vi "ReadDiagram.vi"(1 "reference":refnum<vi>) -> (0 "Diagram":T5)   [LabVIEW 2013]
uses:
  <vilib>/Utility/miscctls.llb/LVBoundsTypeDef.ctl
  <vilib>/Utility/miscctls.llb/LVPositionTypeDef.ctl
  <vilib>/Utility/miscctls.llb/LVRectTypeDef.ctl
  <vilib>/Utility/miscctls.llb/LVBreakpointStatusEnum.ctl
panel:
  out "error out 24":errorcluster
  out "error out 23":errorcluster
  out "error out 22":errorcluster
  out "error out 21":errorcluster
  out "error out 20":errorcluster
  out "error out 19":errorcluster
  out "error out 18":errorcluster
  out "error out 17":errorcluster
  out "error out 16":errorcluster
  out "error out 15":errorcluster
  out "error out 14":errorcluster
  out "error out 13":errorcluster
  out "error out 12":errorcluster
  out "error out 11":errorcluster
  out "error out 10":errorcluster
  out "error out 9":errorcluster
  out "error out 8":errorcluster
  out "error out 7":errorcluster
  out "error out 6":errorcluster
  out "error out 5":errorcluster
  out "error out 4":errorcluster
  out "error out 3":errorcluster
  out "error out 2":errorcluster
  out "error out":errorcluster
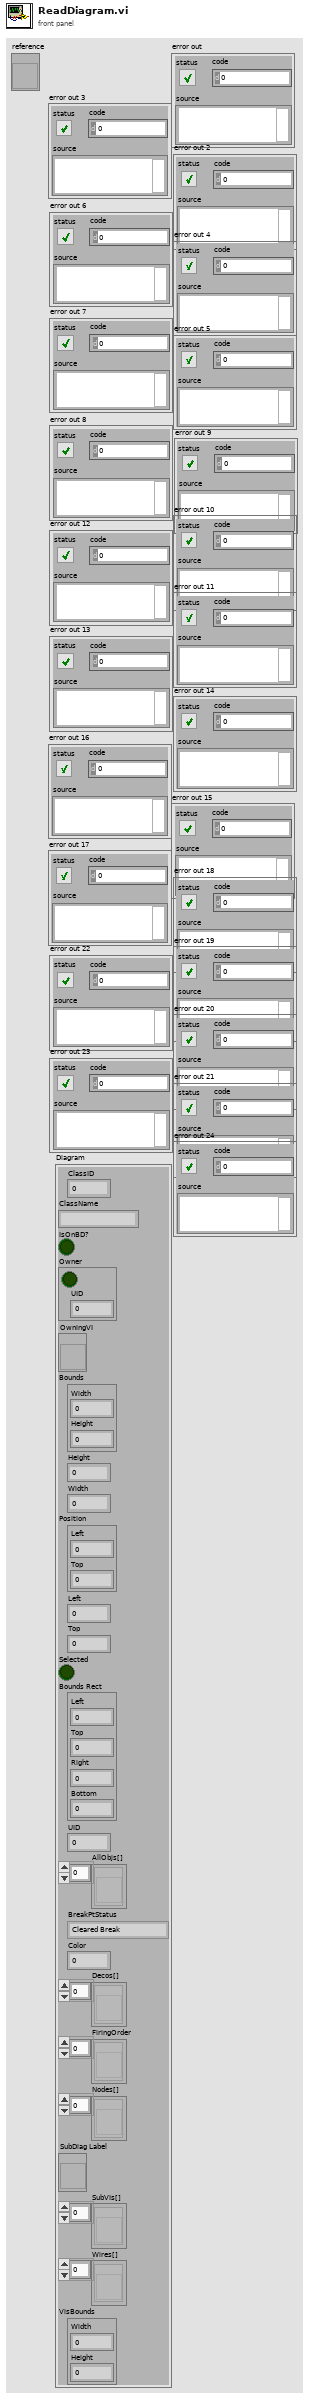
[diagram p1: front panel]
types:
  T1 = typedef "LVBoundsTypeDef.ctl" = cluster{"Width":u32, "Height":u32}
  T2 = typedef "LVPositionTypeDef.ctl" = cluster{"Left":i32, "Top":i32}
  T3 = typedef "LVRectTypeDef.ctl" = cluster{"Left":i16, "Top":i16, "Right":i16, "Bottom":i16}
  T4 = typedef "LVBreakpointStatusEnum.ctl" = enum8{"Cleared Break", "Enabled Break", "Disabled Break"}
  T5 = cluster{"ClassID":u32, "ClassName":string, "IsOnBD?":bool, "Owner":cluster{bool, "UID":i32}, "OwningVI":refnum<vi>, "Bounds":T1, "Height":u32, "Width":u32, "Position":T2, "Left":i32, "Top":i32, "Selected":bool, "Bounds Rect":T3, "UID":i32, "AllObjs[]":refnum<vi>[], "BreakPtStatus":T4, "Color":u32, "Decos[]":refnum<vi>[], "FiringOrder":refnum<vi>[], "Nodes[]":refnum<vi>[], "SubDiag Label":refnum<vi>, "SubVIs[]":refnum<vi>[], "Wires[]":refnum<vi>[], "VisBounds":T1}
  T6 = cluster{"ClassID":u32, "ClassName":string, "IsOnBD?":bool, "Cluster":cluster{bool, "UID":i32}, "OwningVI":refnum<vi>, "Bounds":T1, "Height":u32, "Width":u32, "Position":T2, "Left":i32, "Top":i32, "Selected":bool, "Bounds Rect":T3, "UID":i32, "AllObjs[]":refnum<vi>[], "BreakPtStatus":T4, "Color":u32, "Decos[]":refnum<vi>[], "FiringOrder":refnum<vi>[], "Nodes[]":refnum<vi>[], "SubDiag Label":refnum<vi>, "SubVIs[]":refnum<vi>[], "Wires[]":refnum<vi>[], "VisBounds":T1}
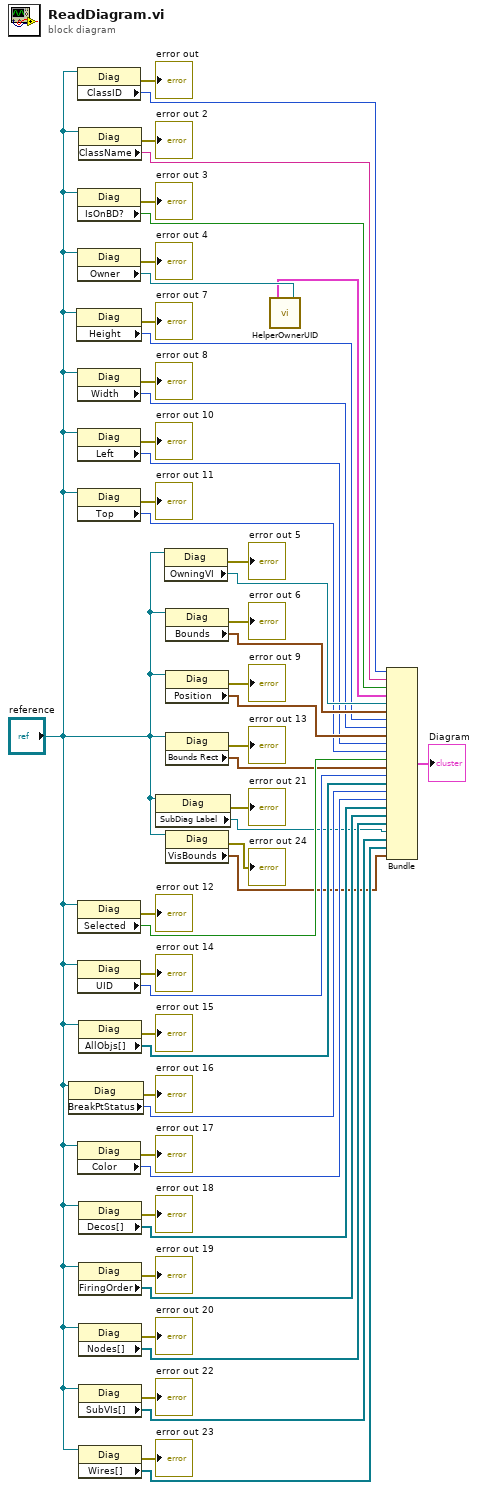
[diagram p0: block diagram]
diagram:
  n1 = property class="Diag"(reference="reference") -> (error out=→"error out 16":errorcluster, "BreakPtStatus"=w18:T4)  [unwired: 1 in, 1 out]
  n2 = property class="Diag"(reference="reference") -> (error out=→"error out 7":errorcluster, "Height"=w36:u32)  [unwired: 1 in, 1 out]
  n3 = property class="Diag"(reference="reference") -> (error out=→"error out":errorcluster, "ClassID"=w49:u32)  [unwired: 1 in, 1 out]
  n4 = property class="Diag"(reference="reference") -> (error out=→"error out 3":errorcluster, "IsOnBD?"=w45:bool)  [unwired: 1 in, 1 out]
  n5 = property class="Diag"(reference="reference") -> (error out=→"error out 4":errorcluster, "Owner"=w43:refnum<vi>)  [unwired: 1 in, 1 out]
  n6 = property class="Diag"(reference="reference") -> (error out=→"error out 8":errorcluster, "Width"=w34:u32)  [unwired: 1 in, 1 out]
  n7 = property class="Diag"(reference="reference") -> (error out=→"error out 10":errorcluster, "Left"=w30:i32)  [unwired: 1 in, 1 out]
  n8 = property class="Diag"(reference="reference") -> (error out=→"error out 11":errorcluster, "Top"=w28:i32)  [unwired: 1 in, 1 out]
  n9 = property class="Diag"(reference="reference") -> (error out=→"error out 12":errorcluster, "Selected"=w26:bool)  [unwired: 1 in, 1 out]
  n10 = property class="Diag"(reference="reference") -> (error out=→"error out 14":errorcluster, "UID"=w22:i32)  [unwired: 1 in, 1 out]
  n11 = property class="Diag"(reference="reference") -> (error out=→"error out 17":errorcluster, "Color"=w16:u32)  [unwired: 1 in, 1 out]
  n12 = property class="Diag"(reference="reference") -> (error out=→"error out 2":errorcluster, "ClassName"=w47:string)  [unwired: 1 in, 1 out]
  n13 = property class="Diag"(reference="reference") -> (error out=→"error out 15":errorcluster, "AllObjs[]"=w20:refnum<vi>[])  [unwired: 1 in, 1 out]
  n14 = property class="Diag"(reference="reference") -> (error out=→"error out 18":errorcluster, "Decos[]"=w14:refnum<vi>[])  [unwired: 1 in, 1 out]
  n15 = property class="Diag"(reference="reference") -> (error out=→"error out 19":errorcluster, "FiringOrder"=w12:refnum<vi>[])  [unwired: 1 in, 1 out]
  n16 = property class="Diag"(reference="reference") -> (error out=→"error out 20":errorcluster, "Nodes[]"=w10:refnum<vi>[])  [unwired: 1 in, 1 out]
  n17 = property class="Diag"(reference="reference") -> (error out=→"error out 22":errorcluster, "SubVIs[]"=w6:refnum<vi>[])  [unwired: 1 in, 1 out]
  n18 = property class="Diag"(reference="reference") -> (error out=→"error out 23":errorcluster, "Wires[]"=w4:refnum<vi>[])  [unwired: 1 in, 1 out]
  n19 = property class="Diag"(reference="reference") -> (error out=→"error out 21":errorcluster, "SubDiag Label"=w8:refnum<vi>)  [unwired: 1 in, 1 out]
  n20 = property class="Diag"(reference="reference") -> (error out=→"error out 5":errorcluster, "OwningVI"=w40:refnum<vi>)  [unwired: 1 in, 1 out]
  n21 = property class="Diag"(reference="reference") -> (error out=→"error out 6":errorcluster, "Bounds"=w38:T1)  [unwired: 1 in, 1 out]
  n22 = property class="Diag"(reference="reference") -> (error out=→"error out 9":errorcluster, "Position"=w32:T2)  [unwired: 1 in, 1 out]
  n23 = property class="Diag"(reference="reference") -> (error out=→"error out 13":errorcluster, "Bounds Rect"=w24:T3)  [unwired: 1 in, 1 out]
  n24 = property class="Diag"(reference="reference") -> (error out=→"error out 24":errorcluster, "VisBounds"=w2:T1)  [unwired: 1 in, 1 out]
  n25 = call "HelperOwnerUID.vi"("Generic in"=w43) -> ("Cluster"=w42:cluster{bool, "UID":i32})
  n26 = Bundle("ClassID"=w49, "ClassName"=w47, "IsOnBD?"=w45, "Cluster"=w42, "OwningVI"=w40, "Bounds"=w38, "Height"=w36, "Width"=w34, "Position"=w32, "Left"=w30, "Top"=w28, "Selected"=w26, "Bounds Rect"=w24, "UID"=w22, "AllObjs[]"=w20, "BreakPtStatus"=w18, "Color"=w16, "Decos[]"=w14, "FiringOrder"=w12, "Nodes[]"=w10, "SubDiag Label"=w8, "SubVIs[]"=w6, "Wires[]"=w4, "VisBounds"=w2) -> (→"Diagram":T6)  [unwired: 1 in]
